vi "ADC_get_array.vi"(3 "Fast sequence size":u32, 4 "Inst_parameter":T1) -> (0 "measures":sgl[][](array[numeric]), 1 "Inst_parameter out":T1)   [LabVIEW 2013]
uses:
  <vilib>/DAQmx/read.llb/DAQmx Read (Analog 2D DBL NChan NSamp).vi
  <vilib>/DAQmx/miscellaneous.llb/DAQmx Fill In Error Info.vi
  <resource>/objmgr/daqmx.rc
panel:
  in  "Emergency stop":bool
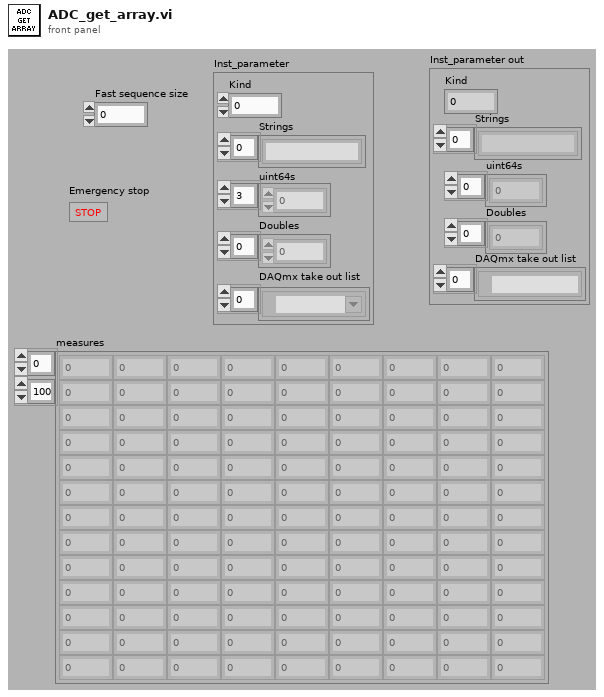
[diagram p1: front panel]
types:
  T1 = cluster{"Kind":u16, "Strings":string[], "uint64s":u64[], "Doubles":dbl[], "DAQmx take out list":refnum<k21>[]}
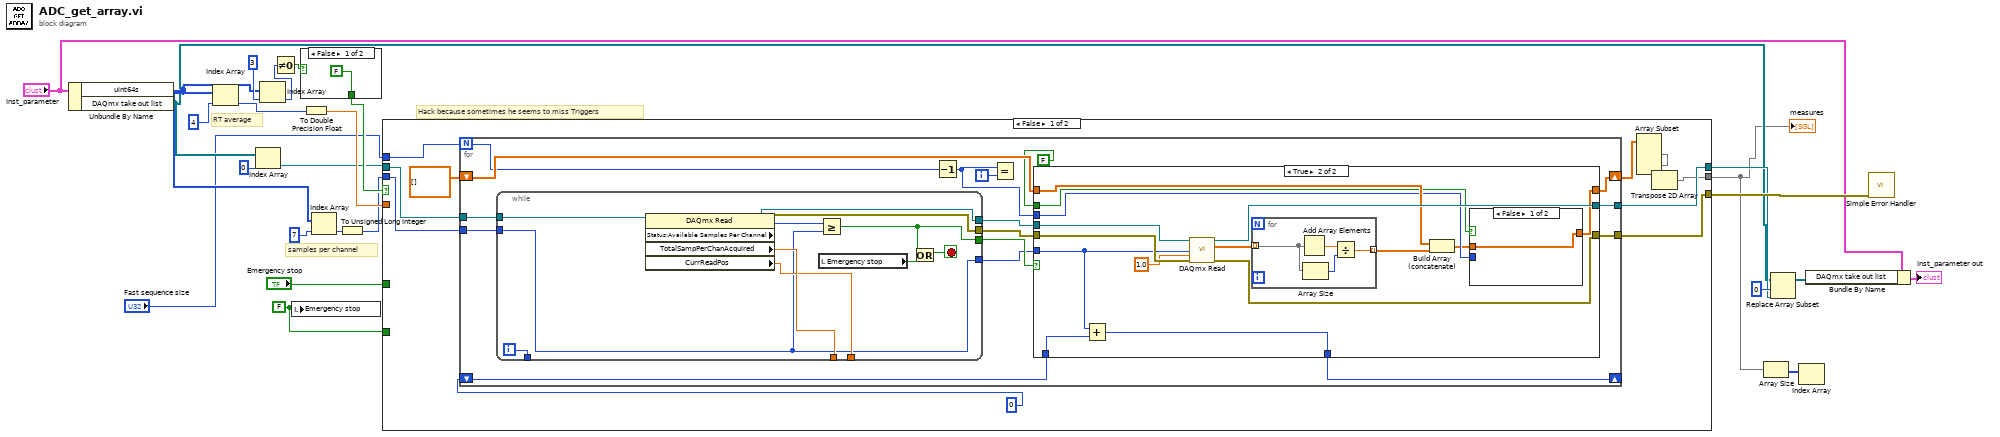
[diagram p0: block diagram]
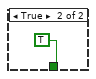
[diagram p2: hidden frame]
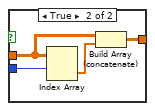
[diagram p4: hidden frame]
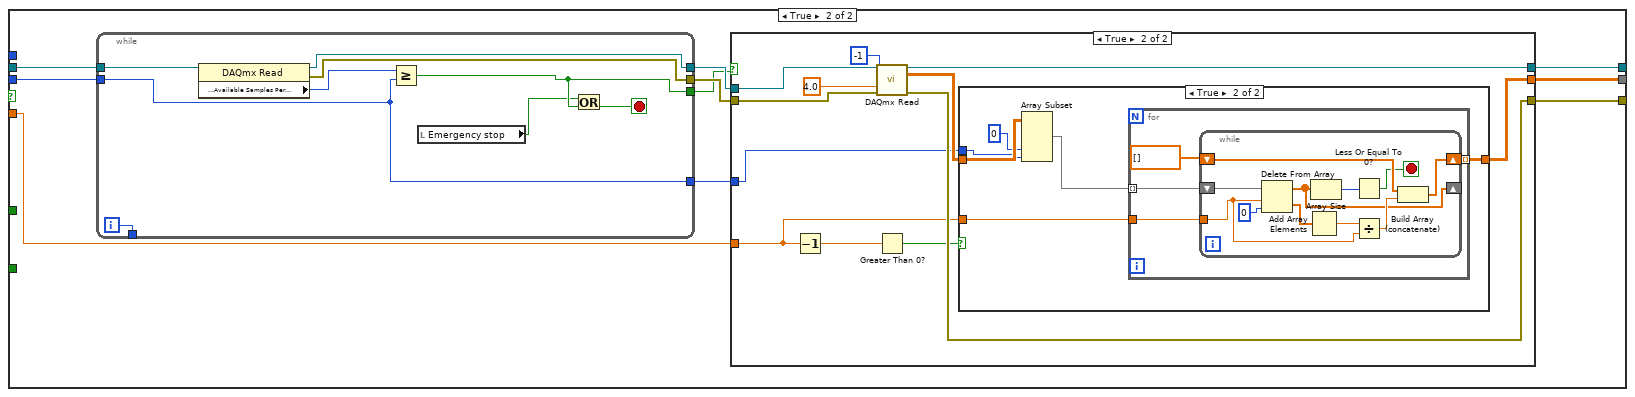
[diagram p5: hidden frame]
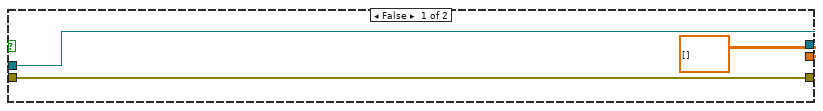
[diagram p6: hidden frame]
diagram:
  w4 = FALSE
  # "samples per channel"
  # "RT average"
  # "Hack because sometimes he seems to miss Triggers"
  n1 = Unbundle By Name("Inst_parameter") -> ("uint64s"=w15:u64[], "DAQmx take out list"=w7:refnum<k21>[])
  n2 = Index Array(array=w15, index=4) -> (element=w23:u64)
  n3 = Index Array(array=w7, index=0) -> (element=w12:refnum<k21>)
  n4 = Index Array(array=w15, index=3) -> (element=w19:u64)
  n5 = Not Equal To 0?(x=w19) -> (x != 0?=w20:bool)
  n6 = local write "Emergency stop"(w4) -> ()
  n7 = case shown="False" w20 {
    tunnel: [FALSE TRUE] -> w18
    frame False {
    }
    frame True {
    }
  }
  n8 = To Double Precision Float(number=w23) -> (double precision float=w22:dbl)
  n9 = Index Array(array=w15, index=7) -> (element=w16:u64)
  n10 = To Unsigned Long Integer(number=w16) -> (unsigned 32bit integer=w14:u32)
  n11 = case shown="False" w18 {
    tunnel: w12 -> [w37 w102]
    tunnel: w14 -> [w36 w101]
    tunnel: [w32 w94] -> w1
    tunnel: "Fast sequence size" -> [w29 _]
    tunnel: [w34 w96] -> w25
    tunnel: [w33 w97] -> w8
    tunnel: w22 -> [_ w95]
    tunnel: "Emergency stop" -> [_ _]
    tunnel: w4 -> [_ _]
    frame False {
      n12 = for {
        N: w29 -> [w43]
        tunnel: w37 -> [w51]
        tunnel: [w50] -> w33
        tunnel: [w49] -> w34
        shift-right: [w41] -> w31
        shift-left: dbl[][] [] -> [w48]
        tunnel: w36 -> [w46]
        shift-right: [w38] -> _
        shift-left: 0 -> [w39]
        i -> [w44]
        n13 = while {
          tunnel: w51 -> [w84]
          tunnel: [w91] -> w53
          tunnel: [w90] -> w52
          tunnel: [w89] -> w47
          tunnel: w46 -> [w82]
          tunnel: [w82] -> w45
          tunnel: [w86] -> _
          tunnel: [w85] -> _
          tunnel: [w83] -> _
          i -> [w86]
          stop <- w88 stop-if-true
          n14 = property class="DAQmx Read"(reference=w84) -> (reference out=w91:refnum<k21>, error out=w90:errorcluster, "Status:Available Samples Per Channel"=w92:u32, "TotalSampPerChanAcquired"=w85:dbl, "CurrReadPos"=w83:dbl)  [unwired: 1 in]
          n15 = Greater Or Equal?(x=w92, y=w82) -> (x >= y?=w89:bool)
          n16 = local read "Emergency stop"() -> (w87:bool)
          n17 = Or(x=w89, y=w87) -> (x .or. y?=w88:bool)
        }
        n18 = Decrement(x=w43) -> (x-1=w42:i32)
        n19 = Equal?(x=w42, y=w44) -> ()  [unwired: 1 out]
        n20 = case shown="True" w47 {
          tunnel: w53 -> [w57 w72]
          tunnel: w52 -> [w56 w71]
          tunnel: [w55 w61] -> w41
          tunnel: [w57 w69] -> w50
          tunnel: [w56 w68] -> w49
          tunnel: w48 -> [w55 w67]
          tunnel: w45 -> [_ w59]
          tunnel: FALSE -> [_ w64]
          tunnel: w42 -> [_ w63]
          tunnel: w39 -> [w54 w60]
          tunnel: [w54 w58] -> w38
          frame False {
          }
          frame True {
            n21 = Add(x=w59, y=w60) -> (x+y=w58:u32)
            n22 = call-poly <vilib>:"DAQmx Read.vi"("task/channels in"=w72, "number of samples per channel"=w59, "timeout"=1.0, "error in"=w71) -> ("task out"=w69:refnum<k21>, "data"=w66:dbl[][], "error out"=w68:errorcluster)  [unwired: 9 out]
            n23 = for {
              tunnel: [w78] -> w65 mode=indexing
              tunnel: w66 -> [w79] mode=indexing
              n24 = Add Array Elements(numeric array=w79) -> (sum=w80:dbl)
              n25 = Array Size(array=w79) -> (size(s)=w81:i32)
              n26 = Divide(x=w80, y=w81) -> (x/y=w78:dbl)
            }
            n27 = Build Array (concatenate)(w67, w65) -> (w62:dbl[][])
            n28 = case shown="False" w64 {
              tunnel: w63 -> [_ w74]
              tunnel: w62 -> [w73 w76]
              tunnel: [w73 w75] -> w61
              frame False {
              }
              frame True {
                n29 = Index Array(array=w76, index (row)=w74) -> (element=w77:dbl[])  [unwired: 1 in]
                n30 = Build Array (concatenate)(w76, w77) -> (w75:dbl[][])
              }
            }
          }
        }
      }
      n31 = Array Subset(array=w31) -> (w30:dbl[][])  [unwired: 4 in]
      n32 = Transpose 2D Array(2D array=w30) -> (transposed array=w32:dbl[][])
    }
    frame True {
      n33 = while {
        tunnel: w102 -> [w147]
        tunnel: [w146] -> w99
        tunnel: [w145] -> w100
        tunnel: [w144] -> w98
        tunnel: w101 -> [w141]
        tunnel: [w141] -> w93
        tunnel: [w140] -> _
        i -> [w140]
        stop <- w143 stop-if-true
        n34 = property class="DAQmx Read"(reference=w147) -> (reference out=w146:refnum<k21>, error out=w145:errorcluster, "Status:Available Samples Per Channel"=w148:u32)  [unwired: 1 in]
        n35 = Greater Or Equal?(x=w148, y=w141) -> (x >= y?=w144:bool)
        n36 = local read "Emergency stop"() -> (w142:bool)
        n37 = Or(x=w142, y=w144) -> (x .or. y?=w143:bool)
      }
      n38 = case shown="True" w98 {
        tunnel: w99 -> [w105 w117]
        tunnel: w100 -> [w104 w116]
        tunnel: [dbl[][] [] w111] -> w94
        tunnel: [w105 w114] -> w97
        tunnel: [w104 w113] -> w96
        tunnel: w95 -> [_ w110]
        tunnel: w93 -> [_ w106]
        frame False {
        }
        frame True {
          n39 = Decrement(x=w110) -> (x-1=w109:dbl)
          n40 = call-poly <vilib>:"DAQmx Read.vi"("task/channels in"=w117, "number of samples per channel"=-1, "timeout"=4.0, "error in"=w116) -> ("task out"=w114:refnum<k21>, "data"=w112:dbl[][], "error out"=w113:errorcluster)  [unwired: 9 out]
          n41 = Greater Than 0?(x=w109) -> (x > 0?=w108:bool)
          n42 = case shown="True" w108 {
            tunnel: w112 -> [w118 w122]
            tunnel: w110 -> [_ w124]
            tunnel: [w118 w123] -> w111
            tunnel: w106 -> [_ w120]
            frame False {
            }
            frame True {
              n43 = Array Subset(array=w122, index (col)=0 ("index (row)"), length (col)=w120) -> (w121:dbl[][])  [unwired: 2 in]
              n44 = for {
                tunnel: w121 -> [w128] mode=indexing
                tunnel: w124 -> [w127]
                tunnel: [w126] -> w123 mode=indexing
                n45 = while {
                  tunnel: w127 -> [w129]
                  shift-right: [w134] -> w126
                  shift-left: dbl[] [] -> [w135]
                  shift-right: [w133] -> _
                  shift-left: w128 -> [w139]
                  stop <- w130 stop-if-true
                  n46 = Delete From Array(array=w139, length=w129, index=0 ("index (row)")) -> (deleted portion=w137:dbl[], array with subset deleted=w133:dbl[])
                  n47 = Add Array Elements(numeric array=w137) -> (sum=w131:dbl)
                  n48 = Array Size(array=w133) -> (size(s)=w132:i32)
                  n49 = Less Or Equal To 0?(x=w132) -> (x <= 0?=w130:bool)
                  n50 = Divide(x=w131, y=w129) -> (x/y=w136:dbl)
                  n51 = Build Array (concatenate)(w135, w136) -> (w134:dbl[])
                }
              }
            }
          }
        }
      }
    }
  }
  "measures" <- w1
  n52 = Array Size(array=w1) -> (size(s)=w2:i32[])
  n53 = Replace Array Subset(array=w7, new element=w8, index=0) -> (w10:refnum<k21>[])
  n54 = Index Array(array=w2) -> ()  [unwired: 1 in, 1 out]
  n55 = Bundle By Name(cluster="Inst_parameter", "DAQmx take out list"=w10) -> (→"Inst_parameter out":T1)
  n56 = call <vilib>:"Simple Error Handler.vi"("error in (no error)"=w25) -> ()  [unwired: 4 in, 5 out]
